vi "LDA Conversion factor.vi"(1 "Focal Length":dbl, 2 "Beam Separation (mm)":dbl, 3 "Wavelength (nm)":dbl) -> (0 "cf":dbl format="%#_9f")   [LabVIEW 2021]
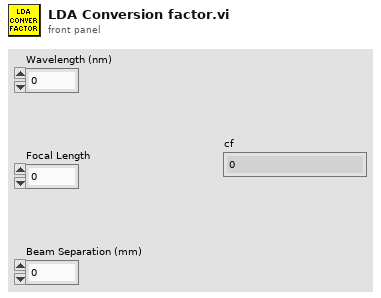
[diagram p1: front panel]
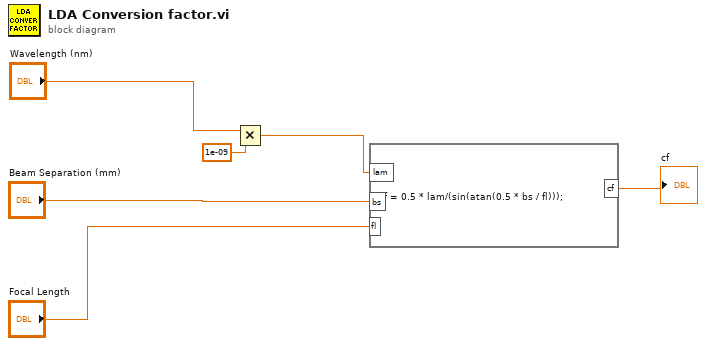
[diagram p0: block diagram]
diagram:
  n1 = Multiply(x="Wavelength (nm)", y=1e-09) -> (x*y=w1:dbl)
  n2 = formula code="cf = 0.5 * lam/(sin(atan(0.5 * bs / fl)));"("bs"="Beam Separation (mm)", "fl"="Focal Length", "lam"=w1) -> ("cf"=→"cf":dbl)
